vi "saf_cdb_update.vi"(8 "Noise":bool[](array[boolean]), 9 "Parameters":T1={"Order"=0, "Time constant"=0.0, "Detrend mode"=enum."Robust linear", "TD amplitude limit"=0.0, "FFT filter"=TRUE, "Notch channels"=[], "LF cutoff"=0, "FD amplitude limit"=0.0}, 10 "Model":cdb[](array[numeric]), 11 "Buffer":cdb[](array[numeric])) -> (3 "New model":cdb[](array[numeric]))   [LabVIEW 2014]
uses:
  averaging_filter_params.ctl
  detrend_mode.ctl
  <vilib>/Analysis/2dsp.llb/Complex FFT.vi
  <vilib>/Analysis/2dsp.llb/Inverse Complex FFT.vi
  <vilib>/Analysis/NI_AALPro.lvlib
panel:
  out "FFT filter":dbl[][](graph)
  # "Debug"
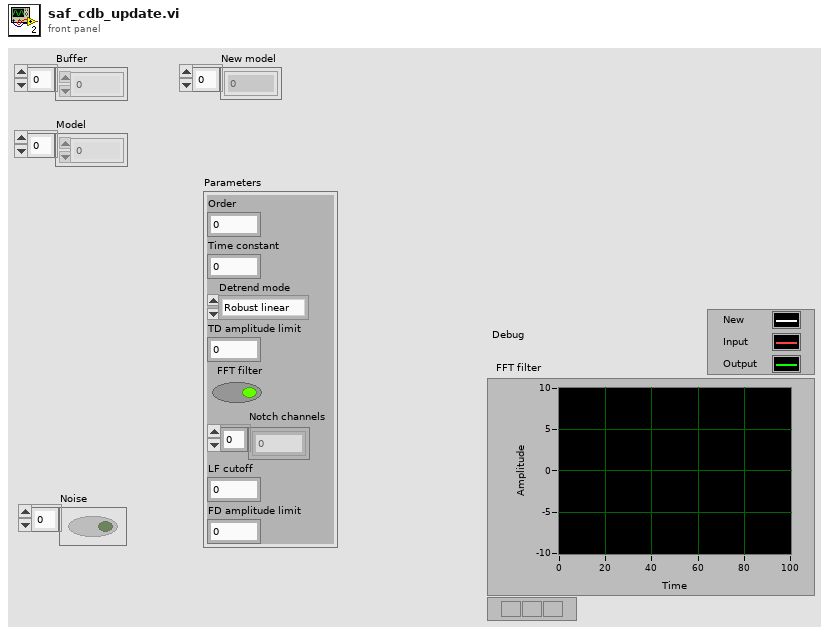
[diagram p1: front panel]
types:
  T1 = typedef "averaging_filter_params.ctl" = cluster{"Order":i32, "Time constant":dbl, "Detrend mode":T2, "TD amplitude limit":dbl, "FFT filter":bool, "Notch channels":i32[], "LF cutoff":i32, "FD amplitude limit":dbl}
  T2 = typedef "detrend_mode.ctl" = enum16{"Zero mean", "Linear", "Robust linear"}
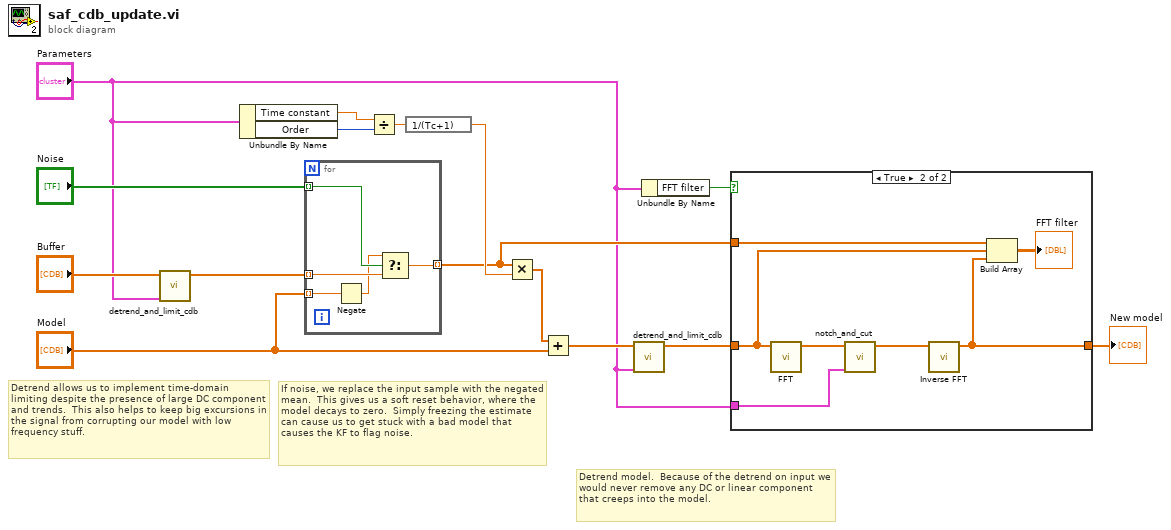
[diagram p0: block diagram]
diagram:
  # "If noise, we replace the input sample with the negated mean.  This gives us a soft reset behavior, where the model decays to zero.  Simply freezing the estimate can cause us to get stuck with a bad model that causes the KF to flag noise."
  # "Detrend allows us to implement time-domain limiting despite the presence of large DC component and trends.  This also helps to keep big excursions in the signal from corrupting our model with low frequency stuff."
  # "Detrend model.  Because of the detrend on input we would never remove any DC or linear component that creeps into the model."
  n1 = call "detrend_and_limit_cdb.vi"("Parameters"="Parameters", "Input"="Buffer") -> ("Output"=w6:cdb[])  [unwired: 9 in]
  n2 = Unbundle By Name("Parameters") -> ("Time constant"=w11:dbl, "Order"=w10:i32)
  n3 = for {
    tunnel: w6 -> [w19] mode=indexing
    tunnel: "Model" -> [w17] mode=indexing
    tunnel: "Noise" -> [w20] mode=indexing
    tunnel: [w18] -> w7 mode=indexing
    n4 = Negate(x=w17) -> (-x=w16:cdb)
    n5 = Select(t=w16, s=w20, f=w19) -> (s? t:f=w18:cdb)
  }
  n6 = Divide(x=w11, y=w10) -> (x/y=w12:dbl)
  n7 = expression code="1/(Tc+1)"(w12) -> (w13:dbl)
  n8 = Multiply(x=w7, y=w13) -> (x*y=w15:cdb[])
  n9 = Add(x=w15, y="Model") -> (x+y=w2:cdb[])
  n10 = call "detrend_and_limit_cdb.vi"("Parameters"="Parameters", "Input"=w2) -> ("Output"=w4:cdb[])  [unwired: 9 in]
  n11 = Unbundle By Name("Parameters") -> ("FFT filter"=w5:bool)
  n12 = case shown="True" w5 {
    tunnel: w4 -> [w21 w28]
    tunnel: [w21 w26] -> w14
    tunnel: w7 -> [_ w23]
    tunnel: "Parameters" -> [_ w22]
    frame False {
    }
    frame True {
      n13 = call-poly <vilib>:"FFT.vi"("X"=w28) -> ("FFT {X}"=w25:cdb[])  [unwired: 9 in, 1 out]
      n14 = call "notch_and_cut.vi"("Parameters"=w22, "In"=w25) -> ("Out"=w24:cdb[])  [unwired: 9 in]
      n15 = call-poly <vilib>:"Inverse FFT.vi"("FFT {X}"=w24) -> ("X"=w26:cdb[])  [unwired: 9 in, 1 out]
      n16 = Build Array(w23, w28, w26) -> (→"FFT filter":cdb[][])
    }
  }
  "New model" <- w14
